vi "Scale Motor Output.vi"(1 "Exponent":dbl, 2 "Error Input":dbl, 3 "Motor Input":u32) -> (0 "Output":u32)   [LabVIEW 2013, in "ProcessorHelperFunctions.lvlib"]
uses:
  ProcessorHelperFunctions.lvlib
panel:
  # "(0 to 512, 255 = stop)"
  # "Positive number"
  # "(0 to 512, 255 = stop)"
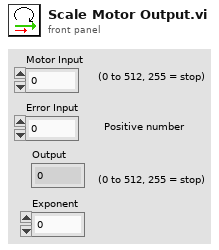
[diagram p1: front panel]
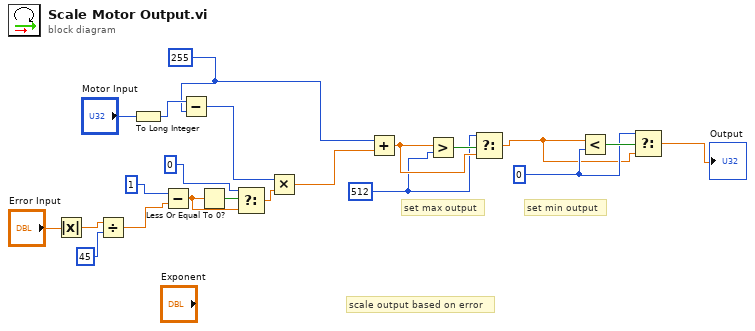
[diagram p0: block diagram]
diagram:
  w11 = 0
  w13 = 512
  w17 = 255
  # "set min output"
  # "set max output"
  # "scale output based on error"
  n1 = Absolute Value(x="Error Input") -> (abs(x)=w6:dbl)
  n2 = Divide(x=w6, y=45) -> (x/y=w7:dbl)
  n3 = To Long Integer(number="Motor Input") -> (32bit integer=w19:i32)
  n4 = Subtract(x=1, y=w7) -> (x-y=w2:dbl)
  n5 = Subtract(x=w19, y=w17) -> (x-y=w18:i32)
  n6 = Less Or Equal To 0?(x=w2) -> (x <= 0?=w3:bool)
  n7 = Select(t=0, s=w3, f=w2) -> (s? t:f=w4:dbl)
  n8 = Multiply(x=w18, y=w4) -> (x*y=w16:dbl)
  n9 = Add(x=w17, y=w16) -> (x+y=w14:dbl)
  n10 = Greater?(x=w14, y=w13) -> (0:w15:bool)
  n11 = Select(t=w13, s=w15, f=w14) -> (s? t:f=w10:dbl)
  n12 = Less?(x=w10, y=w11) -> (x < y?=w12:bool)
  n13 = Select(t=w11, s=w12, f=w10) -> (s? t:f=→"Output":dbl)
